vi "SetWaveformArraySize.vi"(8 "error in (no error)":errorcluster, 11 "WaveformArray In":waveform(dbl)[](array[waveform])) -> (0 "error out":errorcluster, 3 "WaveformArray Out":waveform(dbl)[](array[waveform]))   [LabVIEW 2014, in "FGenPlugins.lvlib" / "NiPxi6733.lvclass"]
uses:
  NiPxi6733.lvclass
  <vilib>/Waveform/WDTOps.llb/WDT Append Waveforms DBL.vi
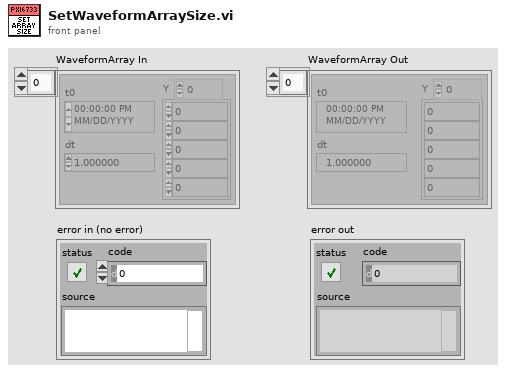
[diagram p1: front panel]
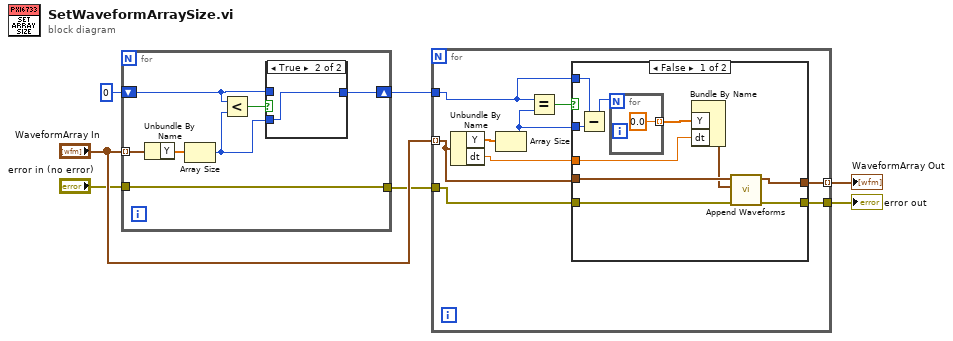
[diagram p0: block diagram]
diagram:
  n1 = for {
    tunnel: "WaveformArray In" -> [w14] mode=indexing
    shift-right: [w10] -> w5
    shift-left: 0 -> [w9]
    tunnel: [w8] -> w3
    tunnel: "error in (no error)" -> [w8]
    n2 = Unbundle By Name(w14) -> ("Y"=w13:dbl[])
    n3 = Array Size(array=w13) -> (size(s)=w11:i32)
    n4 = Less?(x=w9, y=w11) -> (x < y?=w12:bool)
    n5 = case shown="True" w12 {
      tunnel: w11 -> [_ w16]
      tunnel: [w15 w16] -> w10
      tunnel: w9 -> [w15 _]
      frame False {
      }
      frame True {
      }
    }
  }
  n6 = for {
    tunnel: "WaveformArray In" -> [w24] mode=indexing
    tunnel: w5 -> [w22]
    tunnel: w3 -> [w19]
    tunnel: [w23] -> w2 mode=indexing
    tunnel: [w18] -> w1
    n7 = Unbundle By Name(w24) -> ("Y"=w20:dbl[], "dt"=w17:dbl)
    n8 = Array Size(array=w20) -> (size(s)=w21:i32)
    n9 = Equal?(x=w22, y=w21) -> (x = y?=w25:bool)
    n10 = case shown="False" w25 {
      tunnel: w24 -> [w31 w38]
      tunnel: [w29 w38] -> w23
      tunnel: w22 -> [w35 _]
      tunnel: w21 -> [w34 _]
      tunnel: w19 -> [w28 w37]
      tunnel: [w27 w37] -> w18
      tunnel: w17 -> [w26 _]
      frame False {
        n11 = Subtract(x=w35, y=w34) -> (x-y=w33:i32)
        n12 = for {
          N: w33 -> [_]
          tunnel: [0.0] -> w32 mode=indexing
        }
        n13 = Bundle By Name("Y"=w32, "dt"=w26) -> (w30:waveform(dbl))  [unwired: 1 in]
        n14 = call-poly <vilib>:"Append Waveforms.vi"("error in (no error)"=w28, "waveform B"=w30, "waveform A"=w31) -> ("error out"=w27:errorcluster, "waveform out"=w29:waveform(dbl))  [unwired: 7 in]
      }
      frame True {
      }
    }
  }
  "error out" <- w1
  "WaveformArray Out" <- w2
